vi "SSL Detection Frame Simple Estimator Cameras.vi"(4 "IA State Output":T1={"our_robots"=[], "enemy_robots"=[], "balls"=[], "geometry"={"line_width"=0, "field_length"=0, "field_width"=0, "boundary_width"=0, "referee_width"=0, "goal_width"=0, "goal_depth"=0, "goal_wall_width"=0, "center_circle_radius"=0, "defense_radius"=0, "defense_stretch"=0, "free_kick_from_defense_dist"=0, "penalty_spot_from_field_line_dist"=0, "penalty_line_from_spot_dist"=0}, "IA Judge"={"stage"="", "command"="", "our_goalie_id"=0.0, "enemy_goalie_id"=0.0, "command enum"=enum."Halt", "Time"=enum."Azul"}, "Received Timestamp"=timestamp(0 s since 1904-01-01), "Events"={"Touch"=FALSE, "Ball out"=FALSE, "id touch"=0.0, "Ball out of \nVision"=FALSE, "Ball inside \nGoalie area"=FALSE, "Robot not responding"=FALSE, "Robots responding status"=[1.0, 1.0, 1.0, 1.0, 1.0, 1.0], "Enemy Ball \nPossession"=FALSE, "Pass State"=FALSE, "id end of pass"=0.0, "Kick"=FALSE, "Id ini Possession"=0.0, "Ball Possesion"=FALSE, "Id Possesion"=0.0}}, 5 "Estimador":T12, 6 "Time":enum16{"Azul", "Amarelo"}(ring) caption="Enum", 7 "Enable":bool, 8 "ignora esquerda?":bool=TRUE, 9 "ignora lado?":bool=TRUE, 10 "Field Size":T13, 11 "Detection Frame In":T14 {"robots_blue"."height" format="%+4.3f"; "robots_blue"."pixel_y" format="%+4.3f"; "robots_blue"."pixel_x" format="%+4.3f"; "robots_blue"."orientation" format="%+4.3f"; "robots_blue"."y" format="%+4.3f"; "robots_blue"."confidence" format="%4.3f"; "robots_blue"."x" format="%+4.3f"; "robots_yellow"."height" format="%+4.3f"; "robots_yellow"."pixel_y" format="%+4.3f"; "robots_yellow"."pixel_x" format="%+4.3f"; "robots_yellow"."orientation" format="%+4.3f"; "robots_yellow"."y" format="%+4.3f"; "robots_yellow"."confidence" format="%4.3f"; "robots_yellow"."x" format="%+4.3f"}) -> (2 "Field Size Out":T13, 3 "Detection Frame Out":T14 {"robots_blue"."height" format="%+4.3f"; "robots_blue"."pixel_y" format="%+4.3f"; "robots_blue"."pixel_x" format="%+4.3f"; "robots_blue"."orientation" format="%+4.3f"; "robots_blue"."y" format="%+4.3f"; "robots_blue"."confidence" format="%4.3f"; "robots_blue"."x" format="%+4.3f"; "robots_yellow"."height" format="%+4.3f"; "robots_yellow"."pixel_y" format="%+4.3f"; "robots_yellow"."pixel_x" format="%+4.3f"; "robots_yellow"."orientation" format="%+4.3f"; "robots_yellow"."y" format="%+4.3f"; "robots_yellow"."confidence" format="%4.3f"; "robots_yellow"."x" format="%+4.3f"})   [LabVIEW 2017]
uses:
  SSL Detection Frame.ctl
  SSL Detection Robot.ctl
  <vilib>/Analysis/Matrix/Datatypes/RealMatrix.ctl
  SSL Detection Ball.ctl
  Filters/Estimadores.ctl
  Core/AI Input.ctl
  Core/AI Robot.ctl
  Intel/Functions Enum.ctl
  Intel/AttackerStates.ctl
  Path Planning/RRT/PathDests.ctl
  Path Planning/RRT/PathDest.ctl
  Core/AI Ball.ctl
  Core/Field Size.ctl
  Core/AI Judge.ctl
  Intel/Command Enum.ctl
  Events/Events.ctl
  <vilib>/Analysis/Matrix/NI_Matrix.lvlib
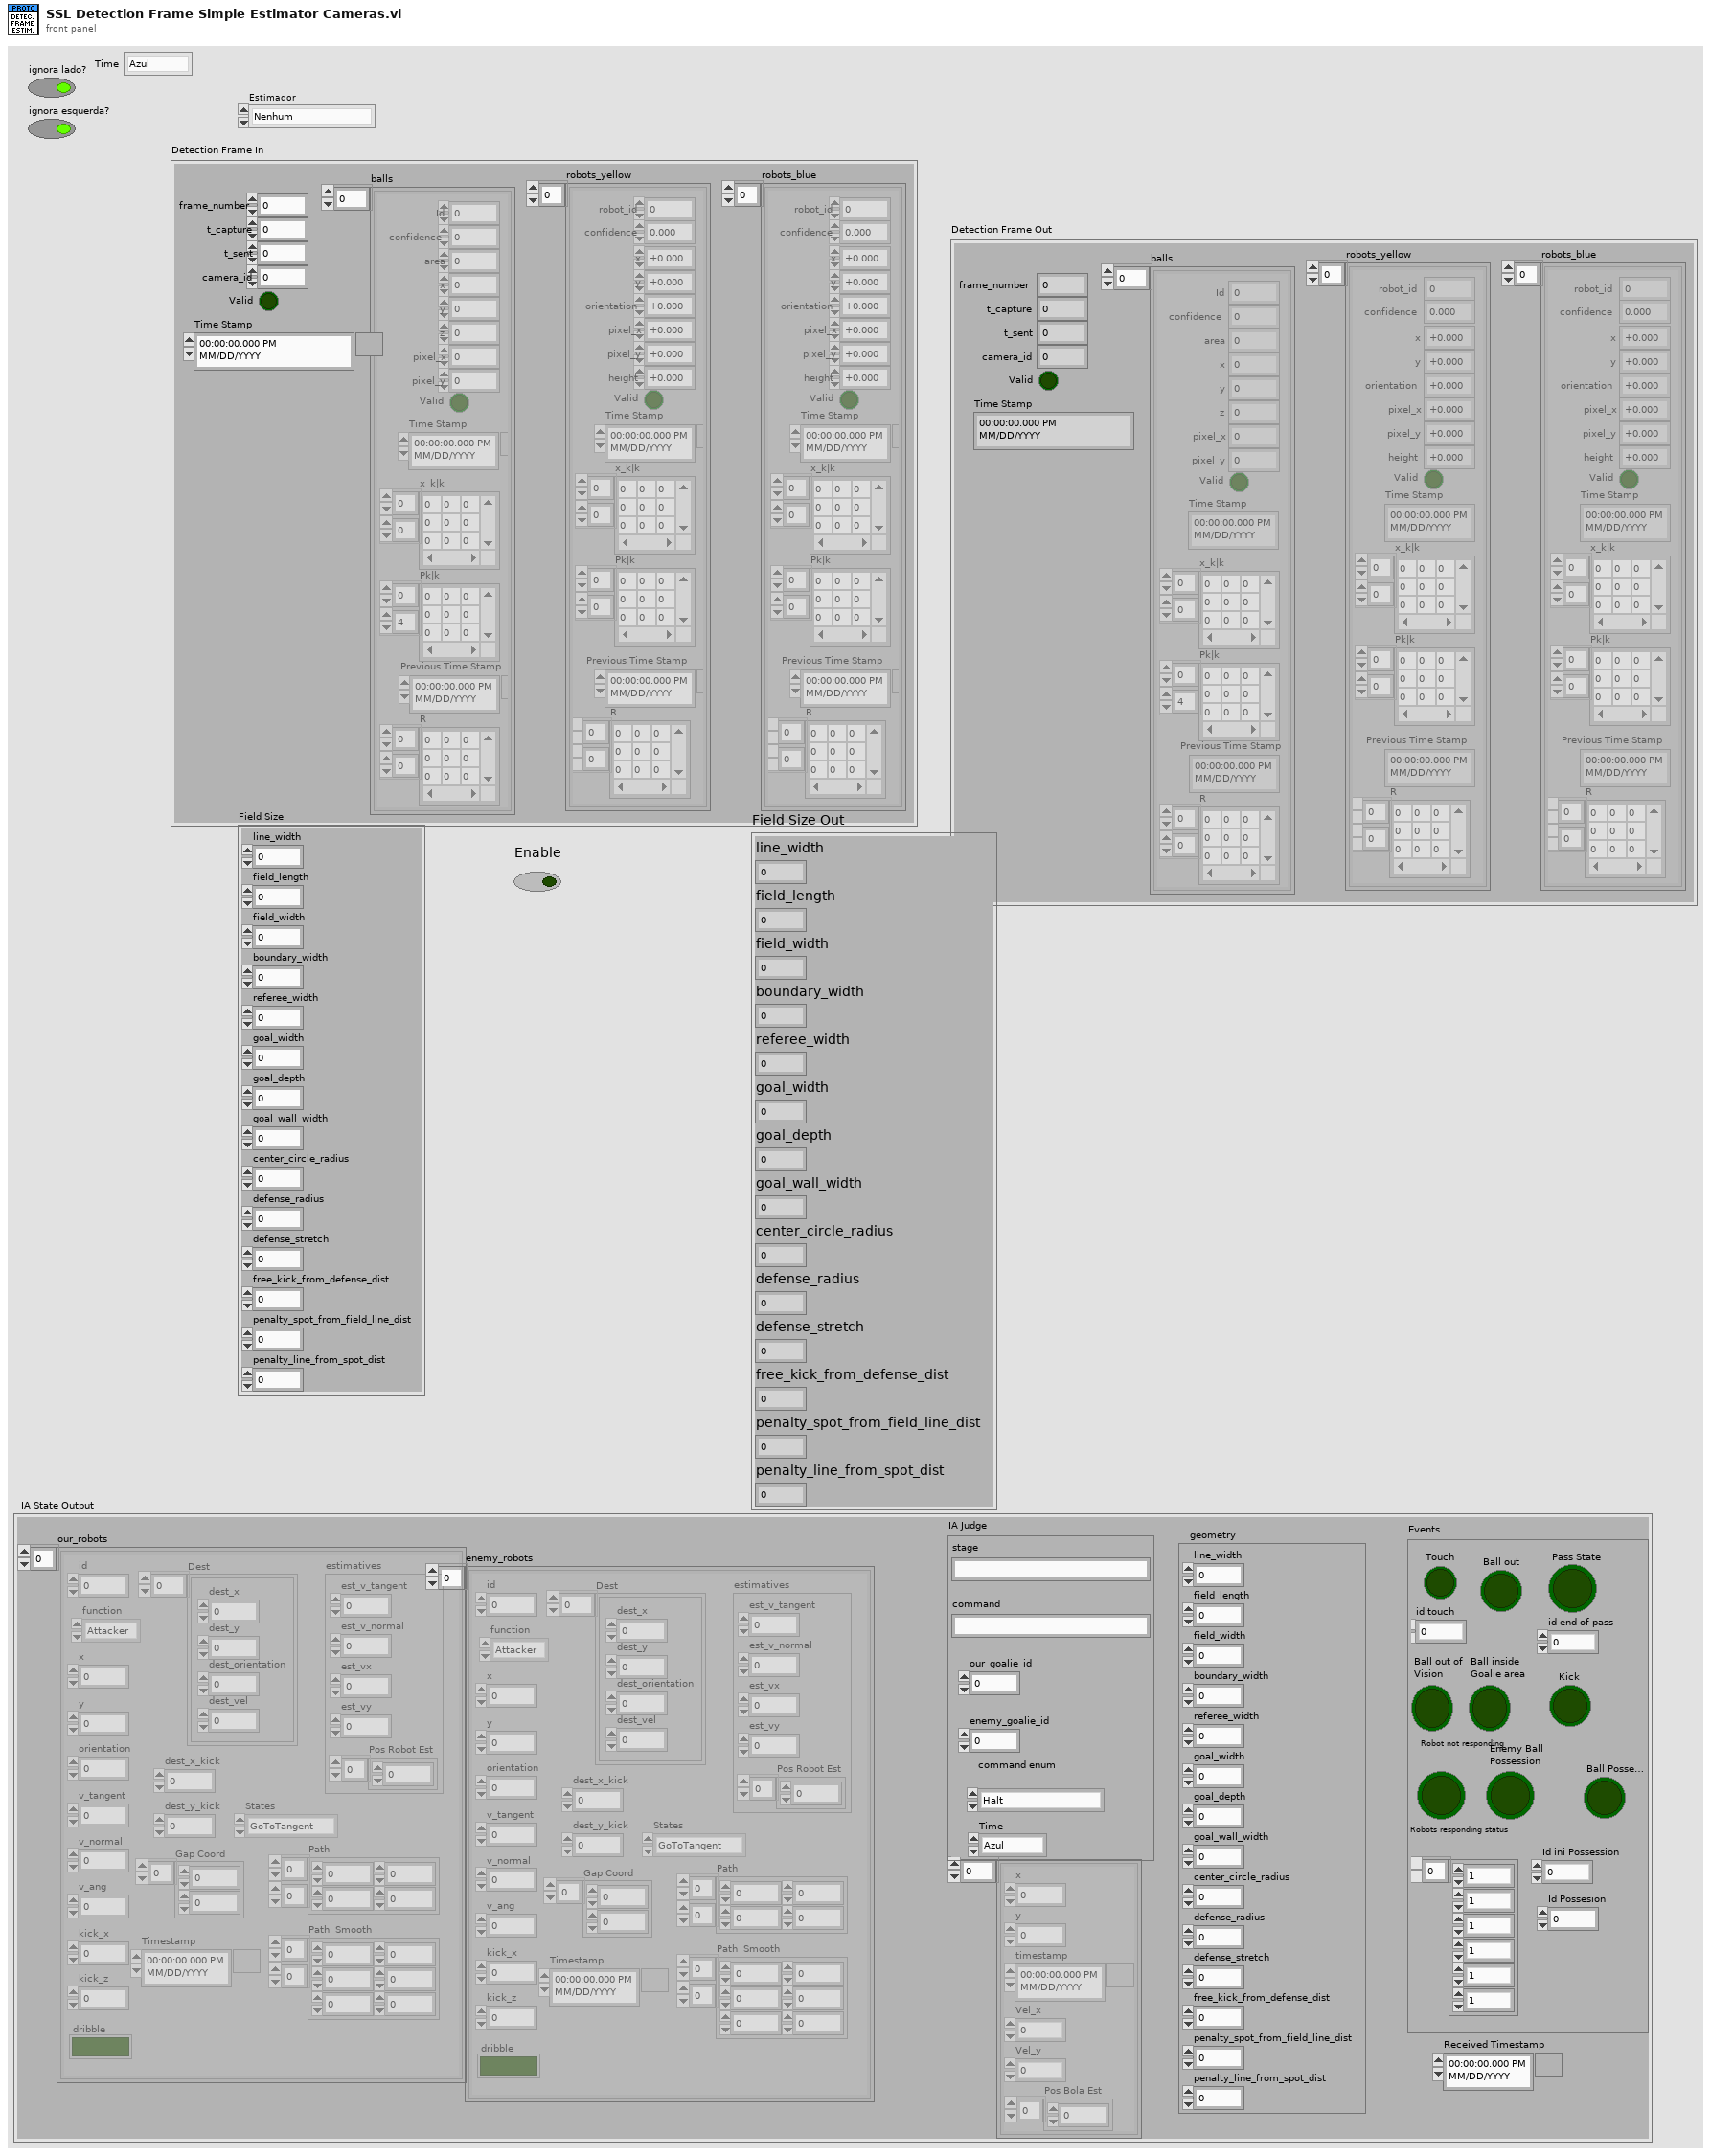
[diagram p1: front panel]
types:
  T1 = typedef "AI Input.ctl" = cluster{"our_robots":T2[], "enemy_robots":T2[], "balls":T7[], "geometry":T8, "IA Judge":T9, "Received Timestamp":timestamp, "Events":T11}
  T2 = typedef "AI Robot.ctl" = cluster{"id":u32, "function":T3, "x":dbl, "y":dbl, "orientation":dbl, "v_tangent":dbl, "v_normal":dbl, "v_ang":dbl, "kick_x":dbl, "kick_z":dbl, "dribble":bool, "Timestamp":timestamp, "estimatives":cluster{"est_v_tangent":dbl, "est_v_normal":dbl, "est_vx":dbl, "est_vy":dbl, "Pos Robot Est":dbl[]}, "dest_x_kick":dbl, "dest_y_kick":dbl, "Gap Coord":dbl[], "States":T4, "Path ":dbl[][], "Path  Smooth":dbl[][], "Dest":T5}
  T3 = typedef "Functions Enum.ctl" = enum16{"Attacker", "Goalie", "Defender", "Striker", "Goto 0", "Dummy", "Kicker", "ZigZag"}
  T4 = typedef "AttackerStates.ctl" = enum16{"Pass", "GoToTangent", "BallGetting", "GoToKick", ""}
  T5 = typedef "PathDests.ctl" = T6[]
  T6 = typedef "PathDest.ctl" = cluster{"dest_x":dbl, "dest_y":dbl, "dest_orientation":dbl, "dest_vel":dbl}
  T7 = typedef "AI Ball.ctl" = cluster{"x":dbl, "y":dbl, "timestamp":timestamp, "Vel_x":dbl, "Vel_y":dbl, "Pos Bola Est":dbl[]}
  T8 = typedef "Field Size.ctl" = cluster{"line_width":u32, "field_length":u32, "field_width":u32, "boundary_width":u32, "referee_width":u32, "goal_width":u32, "goal_depth":u32, "goal_wall_width":u32, "center_circle_radius":u32, "defense_radius":u32, "defense_stretch":u32, "free_kick_from_defense_dist":u32, "penalty_spot_from_field_line_dist":u32, "penalty_line_from_spot_dist":u32}
  T9 = typedef "AI Judge.ctl" = cluster{"stage":string, "command":string, "our_goalie_id":dbl, "enemy_goalie_id":dbl, "command enum":T10, "Time":enum16{"Azul", "Amarelo"}}
  T10 = typedef "Command Enum.ctl" = enum16{"Halt", "Stop", "Force Start", "PKA Normal Start", "Prepare Kickoff Ally", "PKE Normal Start", "Prepare Kickoff Enemy", "Prepare Penalty Ally", "PPA Normal Start", "Prepare Penalty Enemy", "PPE Normal Start", "Direct Free Enemy", "Direct Free Ally", "Indirect Free Enemy", "Indirect Free Ally", "Timeout Enemy", "Timeout Ally", "Goal Enemy", "Goal Ally", "Ball Placement Enemy", "Ball Placement Ally", "Normal Half Time", "Extra Time Break", "Extra Half Time", "None", "Post Game"}
  T11 = typedef "Events.ctl" = cluster{"Touch":bool, "Ball out":bool, "id touch":dbl, "Ball out of \nVision":bool, "Ball inside \nGoalie area":bool, "Robot not responding":bool, "Robots responding status":dbl[], "Enemy Ball \nPossession":bool, "Pass State":bool, "id end of pass":dbl, "Kick":bool, "Id ini Possession":dbl, "Ball Possesion":bool, "Id Possesion":dbl}
  T12 = typedef "Estimadores.ctl" = enum16{"Nenhum", "Simples", "Kalman"}
  T13 = cluster{"line_width":u32, "field_length":u32, "field_width":u32, "boundary_width":u32, "referee_width":u32, "goal_width":u32, "goal_depth":u32, "goal_wall_width":u32, "center_circle_radius":u32, "defense_radius":u32, "defense_stretch":u32, "free_kick_from_defense_dist":u32, "penalty_spot_from_field_line_dist":u32, "penalty_line_from_spot_dist":u32}
  T14 = typedef "SSL Detection Frame.ctl" = cluster{"frame_number":u32, "t_capture":dbl, "t_sent":dbl, "camera_id":u32, "robots_yellow":T15[], "robots_blue":T15[], "balls":T17[], "Valid":bool, "Time Stamp":timestamp}
  T15 = typedef "SSL Detection Robot.ctl" = cluster{"x":sgl, "robot_id":u32, "confidence":sgl, "y":sgl, "orientation":sgl, "pixel_x":sgl, "pixel_y":sgl, "height":sgl, "Valid":bool, "Time Stamp":timestamp, "x_k|k":T16, "Pk|k":T16, "Previous Time Stamp":timestamp, "R":T16}
  T16 = typedef "NI_Matrix.lvlib/RealMatrix.ctl" = dbl[][]
  T17 = typedef "SSL Detection Ball.ctl" = cluster{"x":sgl, "area":u32, "confidence":sgl, "y":sgl, "z":sgl, "pixel_x":sgl, "pixel_y":sgl, "Valid":bool, "Time Stamp":timestamp, "x_k|k":T16, "Pk|k":T16, "Id":u32, "Previous Time Stamp":timestamp, "R":T16}
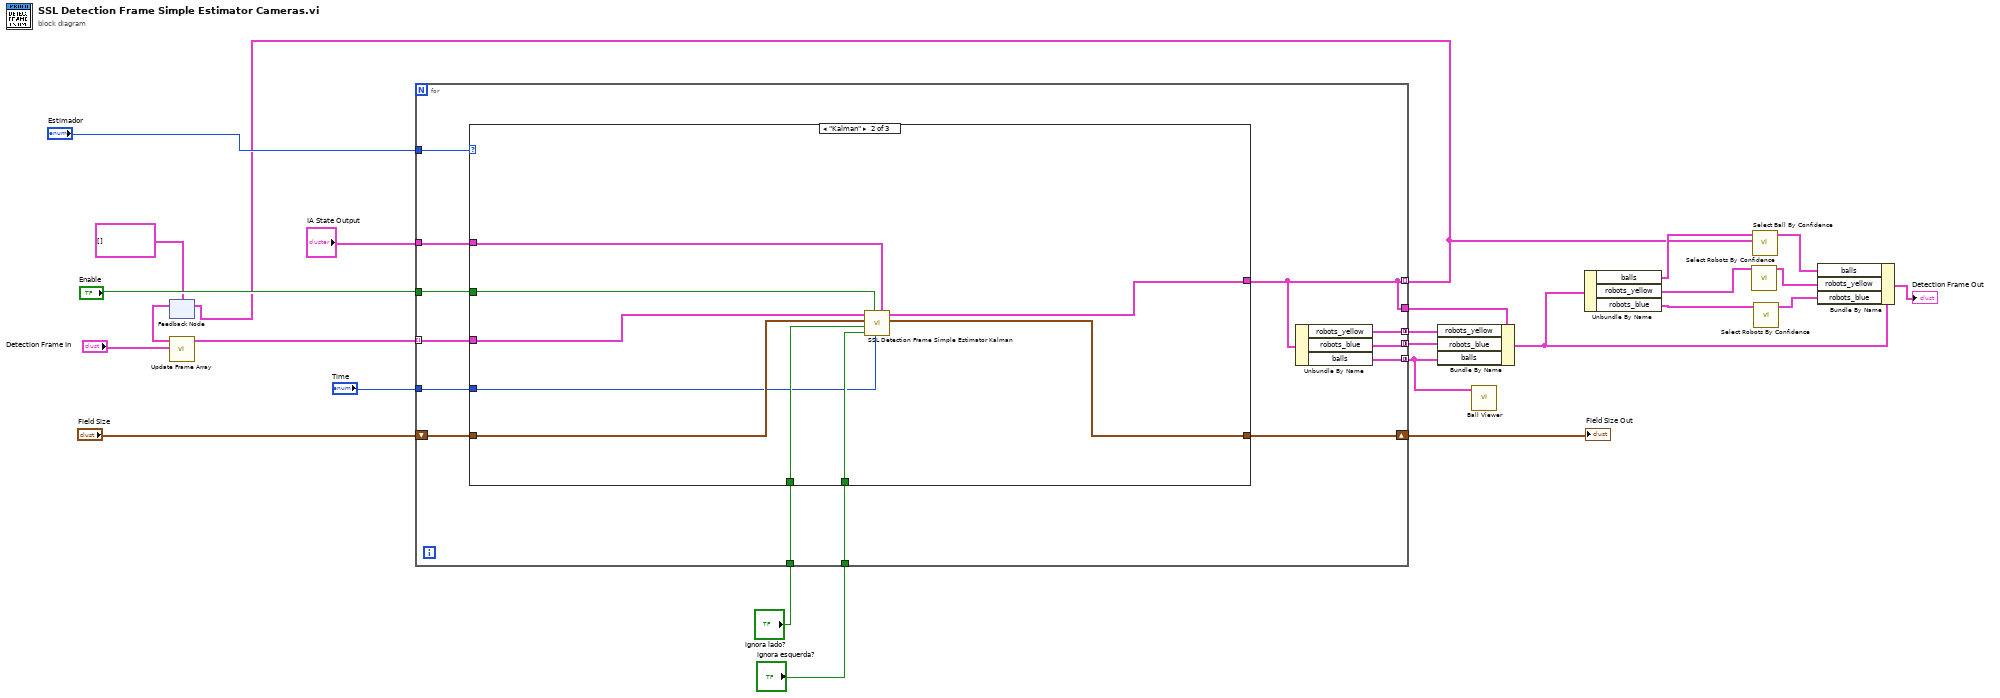
[diagram p0: block diagram]
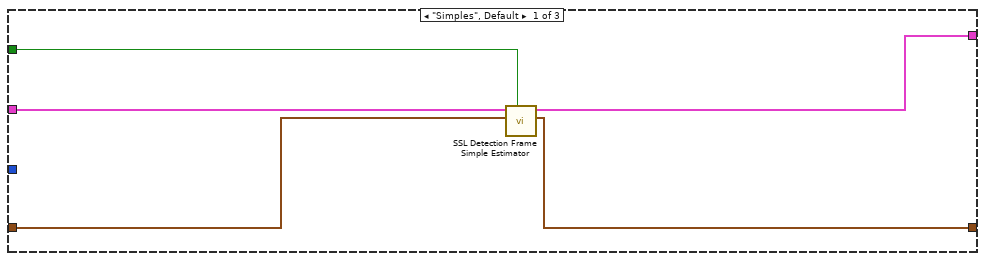
[diagram p2: hidden frame]
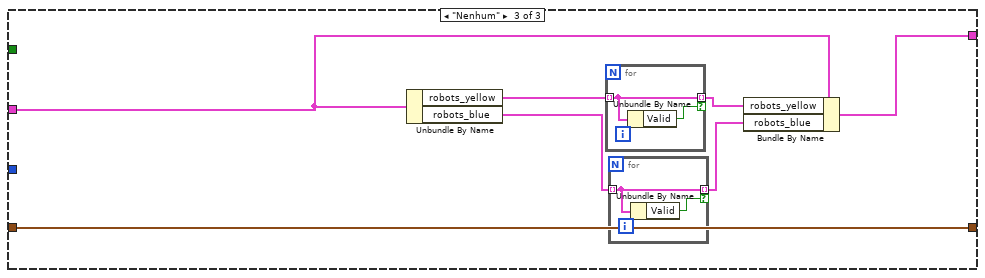
[diagram p3: hidden frame]
diagram:
  n1 = feedback #1(T14[] [] ("Detection Frame In out")) -> (w21:T14[])
  n2 = call "Update Frame Array.vi"("Detection Frame In"="Detection Frame In", "Detection Frame In 2"=w21) -> ("Detection Frame In out"=w22:T14[])  [unwired: 9 in]
  n3 = for {
    tunnel: [w30] -> w3 mode=indexing
    tunnel: "Estimador" -> [w36]
    tunnel: "Enable" -> [w35]
    tunnel: w22 -> [w34] mode=indexing
    shift-right: [w37] -> w24
    shift-left: "Field Size" -> [w38]
    tunnel: [w33] -> w18 mode=concatenating
    tunnel: [w32] -> w17 mode=concatenating
    tunnel: [w31] -> w6 mode=concatenating
    tunnel: [w30] -> w19
    tunnel: "ignora lado?" -> [w29]
    tunnel: "ignora esquerda?" -> [w28]
    tunnel: "Time" -> [w27]
    tunnel: "IA State Output" -> [w26]
    n4 = case shown="\"Kalman\"" w36 {
      tunnel: [w39 w51 w55] -> w30
      tunnel: w34 -> [w43 w52 w57]
      tunnel: w35 -> [w42 w48 _]
      tunnel: w38 -> [w41 w50 w59]
      tunnel: [w40 w49 w59] -> w37
      tunnel: w29 -> [_ w47 _]
      tunnel: w28 -> [_ w46 _]
      tunnel: w27 -> [_ w45 _]
      tunnel: w26 -> [_ w44 _]
      frame "Simples", Default {
        n5 = call "SSL Detection Frame Simple Estimator.vi"("Enable"=w42, "Field Size"=w41, "Detection Frame In"=w43) -> ("Field Size Out"=w40:T13, "Detection Frame Out"=w39:T14)  [unwired: 7 in]
      }
      frame "Kalman" {
        n6 = call "SSL Detection Frame Simple Estimator Kalman.vi"("IA State Output"=w44, "Time"=w45, "Enable"=w48, "ignora esquerda?"=w46, "ignora lado?"=w47, "Field Size"=w50, "Detection Frame In"=w52) -> ("Field Size Out"=w49:T13, "Detection Frame Out"=w51:T14)  [unwired: 3 in]
      }
      frame "Nenhum" {
        n7 = Unbundle By Name(w57) -> ("robots_yellow"=w58:T15[], "robots_blue"=w54:T15[])
        n8 = for {
          tunnel: w58 -> [w63] mode=indexing
          tunnel: [w63] -> w56 mode=indexing if=w62
          n9 = Unbundle By Name(w63) -> ("Valid"=w62:bool)
        }
        n10 = for {
          tunnel: w54 -> [w61] mode=indexing
          tunnel: [w61] -> w53 mode=indexing if=w60
          n11 = Unbundle By Name(w61) -> ("Valid"=w60:bool)
        }
        n12 = Bundle By Name(cluster=w57, "robots_yellow"=w56, "robots_blue"=w53) -> (w55:T14)
      }
    }
    n13 = Unbundle By Name(w30) -> ("robots_yellow"=w33:T15[], "robots_blue"=w32:T15[], "balls"=w31:T17[])
  }
  "Field Size Out" <- w24
  n14 = feedback-in #1(w3) -> ()
  n15 = Bundle By Name(cluster=w19, "robots_yellow"=w18, "robots_blue"=w17, "balls"=w6) -> (w14:T14)
  n16 = call "Ball Viewer.vi"("balls"=w6) -> ()  [unwired: 11 in]
  n17 = Unbundle By Name(w14) -> ("balls"=w5:T17[], "robots_yellow"=w10:T15[], "robots_blue"=w15:T15[])
  n18 = call "Select Robots By Confidence.vi"("robots_blue"=w10) -> ("Array"=w9:T15[])  [unwired: 10 in]
  n19 = call "Select Ball By Confidence.vi"("Array"=w3, "balls"=w5) -> ("balls out"=w4:T17[])  [unwired: 9 in]
  n20 = call "Select Robots By Confidence.vi"("robots_blue"=w15) -> ("Array"=w13:T15[])  [unwired: 10 in]
  n21 = Bundle By Name(cluster=w14, "balls"=w4, "robots_yellow"=w9, "robots_blue"=w13) -> (→"Detection Frame Out":T14)
